vi "test_udp_discovery_server_w-vision.vi"() -> ()   [LabVIEW 2019]
uses:
  <vilib>/userDefined/High Color/IMAQdx.ctl
  <vilib>/vision/driver/NI_Vision_Acquisition_Software.lvlib
  <vilib>/vision/NI_Vision_Development_Module.lvlib
panel:
  out "idx":i32
  out "크기":i32[](array[numeric])
  out "이름":string
  out "Image Pixels (U8) 2":u8[][](array[numeric])
  out "error out 2":errorcluster
  out "Image Pixels (U8)":u8[][](array[numeric])
  out "error out":errorcluster
  out "Image":T1(plugin-control)
  in  "Session In":T2
  out "Client IP Address":string
  in  "stop":bool
  out "n":i32
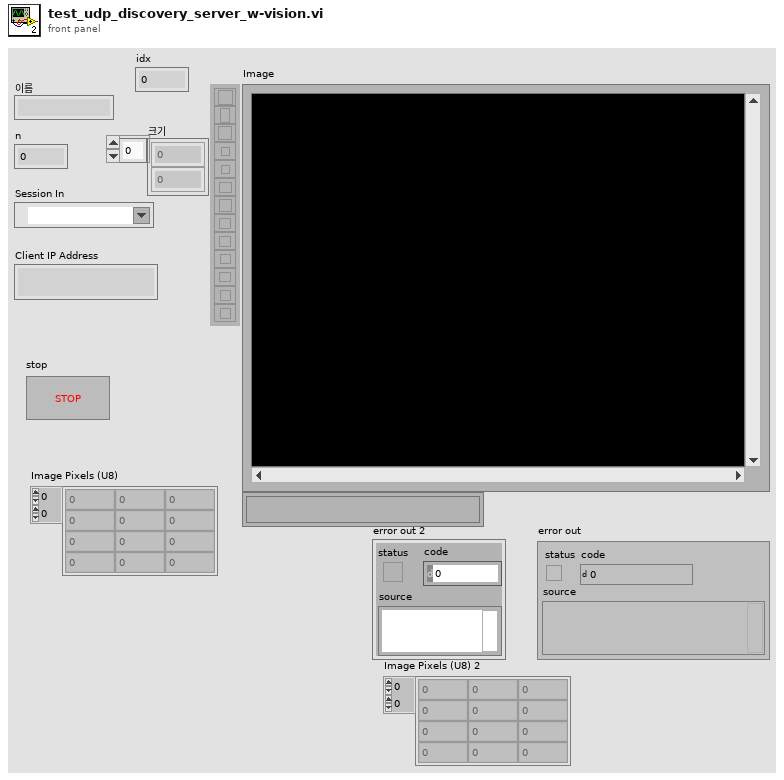
[diagram p1: front panel]
types:
  T1 = typedef "IMAQ Image.ctl" = refnum<image>
  T2 = typedef "IMAQdx.ctl" = refnum<k21>
  T3 = typedef "Image Type" = u32
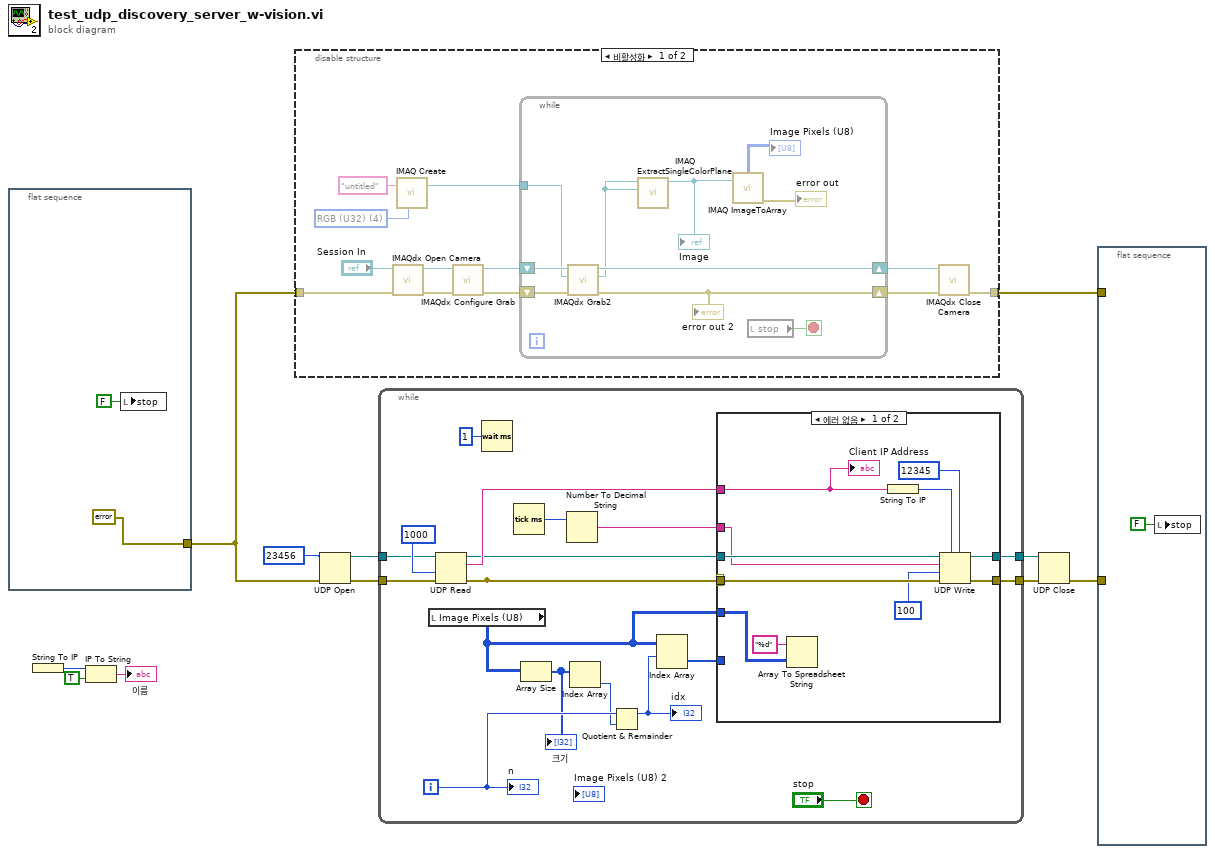
[diagram p0: block diagram]
diagram:
  n1 = flat-sequence {
    tunnel: [errorcluster {"status"=FALSE, "code"=0, "source"=""} ("에러 입력(에러 없음)")] -> w6
    frame #0 {
      n2 = local write "stop"(FALSE ("stop")) -> ()
    }
  }
  n3 = String To IP() -> (0:w3:u32)  [unwired: 1 in]
  n4 = IP To String(1:TRUE ("dot notation? (F)"), 2:w3) -> (0:→"이름":string)
  n5 = disable-structure shown="비활성화" {
    disable-tunnel: w6 -> [w15 _]
    disable-tunnel: [w14 _] -> w5
    frame Disabled {
      w16 = T3 4 items=["Grayscale (U8)", "Grayscale (I16)", "Grayscale (SGL)", "Complex (CSG)", "RGB (U32)", "HSL (U32)", "RGB (U64)", "Grayscale (U16)"] ("Image Type")
      n6 = call <vilib>:"IMAQdx Open Camera.vi"("error in"=w15, "Session In"="Session In") -> ("error out"=w25:errorcluster, "Session Out"=w24:T2)  [unwired: 8 in]
      n7 = call "IMAQ Create"("Image Name"="untitled", "Image Type"=w16) -> ("New Image"=w17:T1)  [unwired: 3 in, 1 out]
      n8 = call <vilib>:"IMAQdx Configure Grab.vi"("error in"=w25, "Session In"=w24) -> ("error out"=w22:errorcluster, "Session Out"=w23:T2)  [unwired: 8 in]
      n9 = while {
        shift-right: [w33] -> w20
        shift-left: w23 -> [w35]
        shift-right: [w31] -> w21
        shift-left: w22 -> [w34]
        tunnel: w17 -> [w32]
        stop <- w26 stop-if-true
        n10 = call <vilib>:"IMAQdx Grab2.vi"("error in"=w34, "Image In"=w32, "Session In"=w35) -> ("error out"=w31:errorcluster, "Image Out"=w28:T1, "Session Out"=w33:T2)  [unwired: 5 in, 1 out]
        "error out 2" <- w31
        n11 = call "IMAQ ExtractSingleColorPlane"("Image Dst"=w28, "Image Src"=w28) -> ("Image Dst Out"=w27:T1)  [unwired: 8 in, 1 out]
        "Image" <- w27
        n12 = call "IMAQ ImageToArray"("Image"=w27) -> ("error out"=→"error out":errorcluster, "Image Pixels (U8)"=→"Image Pixels (U8)":u8[][])  [unwired: 3 in, 3 out]
        n13 = local read "stop"() -> (w26:bool)
      }
      n14 = call <vilib>:"IMAQdx Close Camera.vi"("error in"=w21, "Session In"=w20) -> ("error out"=w14:errorcluster)  [unwired: 9 in]
    }
    frame Enabled {
    }
  }
  n15 = UDP Open(8:w6, 11:u16 23456 ("port")) -> (port=w11:refnum<k16>, 0:w10:errorcluster)  [unwired: 3 in, 1 out]
  n16 = while {
    tunnel: w11 -> [w52]
    tunnel: w10 -> [w51]
    tunnel: [w46] -> w8
    tunnel: [w45] -> w7
    i -> [w42]
    stop <- "stop" stop-if-true
    n17 = local read "Image Pixels (U8)"() -> (w37:u8[][])
    n18 = UDP Read(connection ID=w52, timeout ms (25000)=1000, 8:w51) -> (data out=w50:string, error out=w48:errorcluster, 3:w49:refnum<k16>)  [unwired: 1 in, 2 out]
    n19 = Wait (ms)(milliseconds to wait=u32 1 ("대기 시간 (ms)")) -> ()  [unwired: 1 out]
    n20 = Tick Count (ms)() -> (millisecond timer value=w44:u32)
    n21 = Array Size(array=w37) -> (size(s)=w40:i32[])
    "크기" <- w40
    n22 = Number To Decimal String(number=w44) -> (decimal integer string=w43:string)  [unwired: 1 in]
    n23 = Index Array(array=w40) -> (element=w41:i32)  [unwired: 1 in]
    n24 = Quotient & Remainder(x=w42, y=w41) -> (x-y*floor(x/y)=w39:i32)  [unwired: 1 out]
    "idx" <- w39
    n25 = Index Array(array=w37, index (row)=w39) -> (element=w38:u8[])  [unwired: 1 in]
    n26 = case shown="에러 없음" w48 {
      selector: w48 -> [w61 _]
      tunnel: w50 -> [w58 _]
      tunnel: w49 -> [w62 w65]
      tunnel: w48 -> [_ _]
      tunnel: [w60 w65] -> w46
      tunnel: [w59 _] -> w45
      tunnel: w43 -> [w54 _]
      tunnel: w38 -> [_ _]
      tunnel: w37 -> [w56 _]
      frame No Error {
        n27 = Array To Spreadsheet String(array=w56, 3:"%d" ("포맷 문자열")) -> ()  [unwired: 1 in, 1 out]
        n28 = String To IP(1:w58) -> (0:w63:u32)
        n29 = UDP Write(address=w63, port or service name=u16 12345 ("port"), connection ID=w62, data in=w54, 8:w61, 9:100 ("타임아웃 ms (25000)")) -> (error out=w59:errorcluster, 3:w60:refnum<k16>)
        "Client IP Address" <- w58
      }
      frame Error {
      }
    }
    "n" <- w42
  }
  n30 = UDP Close(connection ID=w8, 8:w7) -> (error out=w4:errorcluster)  [unwired: 1 out]
  n31 = flat-sequence {
    tunnel: w5 -> [_]
    tunnel: w4 -> [_]
    frame #0 {
      n32 = local write "stop"(FALSE ("stop")) -> ()
    }
  }
